vi "Untitled 1.vi"() -> ()   [LabVIEW 2019]
panel:
  out "Execution:State":T1(ring)
  out "Details":string[](array[string])
  out "Errors":string[](array[string])
  out "error out":errorcluster
  out "reference out":refnum<vi>
  in  "Path":path
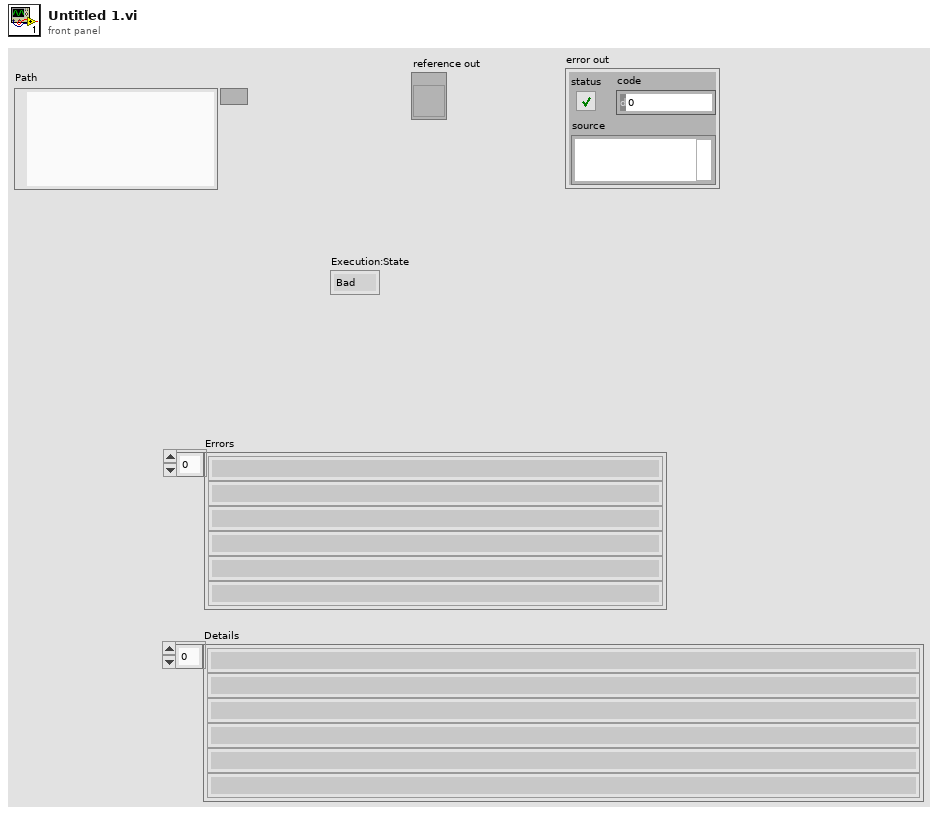
[diagram p1: front panel]
types:
  T1 = enum32{"Bad", "Idle", "Run top level", "Running"}
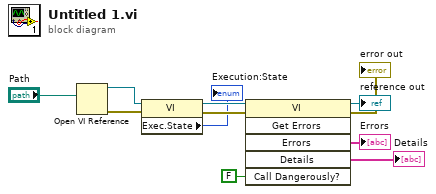
[diagram p0: block diagram]
diagram:
  n1 = Open VI Reference(vi path="Path") -> (vi reference=w10:refnum<vi>, error out=w6:errorcluster)  [unwired: 5 in]
  n2 = property class="VI"(reference=w10, error in=w6) -> (reference out=w9:refnum<vi>, error out=w8:errorcluster, "Exec.State"=→"Execution:State":T1)
  n3 = invoke class="VI" method="Get Errors"(reference=w9, error in=w8, "Call Dangerously?"=FALSE) -> (reference out=→"reference out":refnum<vi>, error out=→"error out":errorcluster, "Errors"=→"Errors":string[], "Details"=→"Details":string[])  [unwired: 3 in, 2 out]
